vi "Confirmation Message - Text--Const.vi"() -> (3 "Message String":string)   [LabVIEW 2017, in "DTacq Plot Display Library.lvlib"]
doc: "Creates a message string, asking the user to confirm the changes."
uses:
  DTacq Plot Display Library.lvlib
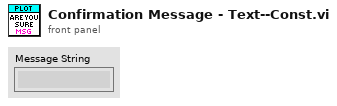
[diagram p1: front panel]
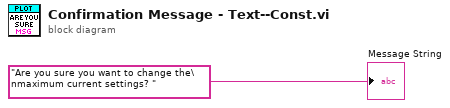
[diagram p0: block diagram]
diagram:
  "Message String" <- "Are you sure you want to change the\nmaximum current settings? " ("message")
